vi "Init.vi"(8 "error in (no error)":errorcluster, 11 "SIM AI Driver in":refnum<class "SIM AI Driver.lvclass">) -> (0 "error out":errorcluster, 3 "SIM AI Driver out":refnum<class "SIM AI Driver.lvclass">)   [LabVIEW 2022 SP3, in "SIM AI Driver.lvclass"]
uses:
  SIM AI Driver.lvclass
  SIM AI Driver.lvclass/SIM AI Driver.ctl
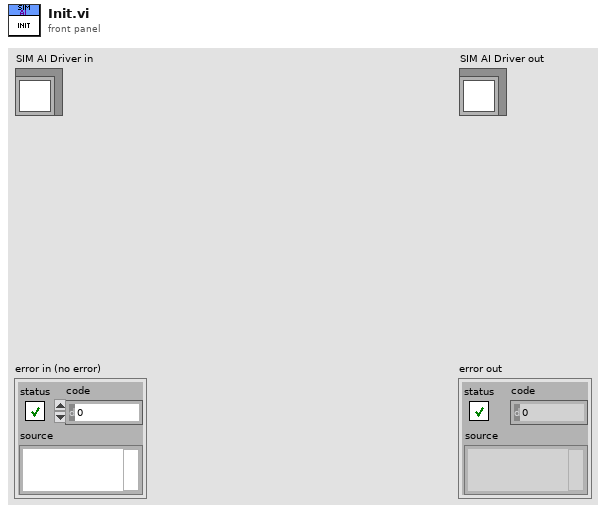
[diagram p1: front panel]
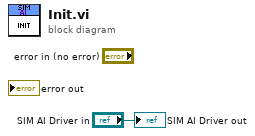
[diagram p0: block diagram]
diagram:
  "SIM AI Driver out" <- "SIM AI Driver in"
